vi "Build Target.vi"   [LabVIEW 2017]
doc: "Builds all components and the VI package for a project/target.\n\nThis VI is called as part of the automated build process. It is configured to run when loaded."
uses:
  <vilib>/AppBuilder/AB_API_Simple/Build (path).vi
  <vilib>/AppBuilder/AB_API_Simple/NI_App_Builder_API.lvlib
  <vilib>/JKI/VIPM API/VIPM API_vipm_api.lvlib
panel:
  # "Overview: Builds all components and the VI package for a project/target\nRequirements: VIPM Pro, VIPM API\nInstructions: Run this VI."
  # "This VI is called as part of the automated build process. It should not be aborted or closed while running. It will build all of the Source Distribution build specifications for the project/target, start VIPM, build the package, then close VIPM and LabVIEW. It is configured to run when called.\n\nThis VI will fail if VIPM Pro and the VIPM API are not installed or available."
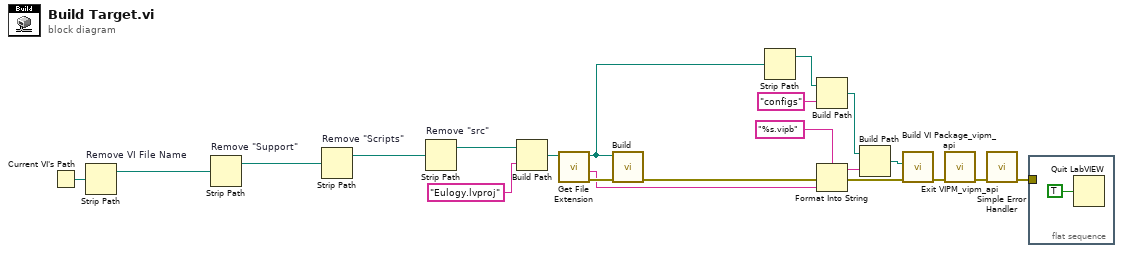
[diagram p0: block diagram]
diagram:
  n1 = Current VI's Path() -> (path=w5:path)
  n2 = Strip Path "Remove VI File Name"(path=w5) -> (stripped path=w11:path)  [unwired: 1 out]
  n3 = Strip Path "Remove \"Support\""(path=w11) -> (stripped path=w10:path)  [unwired: 1 out]
  n4 = Strip Path "Remove \"Scripts\""(path=w10) -> (stripped path=w9:path)  [unwired: 1 out]
  n5 = Strip Path "Remove \"src\""(path=w9) -> (stripped path=w8:path)  [unwired: 1 out]
  n6 = Build Path(base path=w8, name or relative path="Eulogy.lvproj") -> (appended path=w6:path)
  n7 = call <vilib>:"Get File Extension.vi"("file"=w6) -> ("error out"=w16:errorcluster, "filename without extension"=w14:string, "dup file"=w15:path)  [unwired: 6 in, 2 out]
  n8 = call-poly <vilib>:"Build.vi"("error in (no error)"=w16, "Path to project"=w15) -> ("error out"=w21:errorcluster)  [unwired: 8 in, 1 out]
  n9 = Strip Path(path=w15) -> (stripped path=w17:path)  [unwired: 1 out]
  n10 = Build Path(base path=w17, name or relative path="configs") -> (appended path=w19:path)
  n11 = Format Into String(format string="%s.vipb", error in=w21, w14) -> (resulting string=w12:string, error out=w1:errorcluster)  [unwired: 1 in]
  n12 = Build Path(base path=w19, name or relative path=w12) -> (appended path=w18:path)
  n13 = call <vilib>:"Build VI Package_vipm_api.vi"("error in (no error)"=w1, "Path to VIPB File"=w18) -> ("error out"=w4:errorcluster)  [unwired: 8 in, 1 out]
  n14 = call <vilib>:"Exit VIPM_vipm_api.vi"("error in (no error)"=w4) -> ("error out"=w3:errorcluster)  [unwired: 10 in]
  n15 = call <vilib>:"Simple Error Handler.vi"("error in (no error)"=w3) -> ("error out"=w2:errorcluster)  [unwired: 4 in, 4 out]
  n16 = flat-sequence {
    tunnel: w2 -> [_]
    frame #0 {
      n17 = Quit LabVIEW(quit? (T)=TRUE) -> ()
    }
  }
